vi "Change Desired Temperature.vi"(8 "error in (no error)":cluster{"状态":bool, "代码":i32, "源":string} caption="错误输入（无错误）", 10 "待维持的温度":dbl, 11 "冷却器的控制器输入":refnum<class "Cooler Controller.lvclass">) -> (0 "error out":cluster{"状态":bool, "代码":i32, "源":string} caption="错误输出", 3 "冷却器的控制器输出":refnum<class "Cooler Controller.lvclass">)   [LabVIEW 2013, in "Cooler Controller.lvlib" / "Cooler Controller.lvclass"]
doc: "更改冷却系统需要维持的温度。"
uses:
  Cooler Controller.lvclass
  Cooler Controller.lvclass/Cooler Controller.ctl
  Cooler/Write Desired Temperature Msg/Write Desired Temperature Msg.lvclass/Write Desired Temperature Msg.ctl
  <vilib>/ActorFramework/Message Enqueuer/Message Enqueuer.lvclass/Message Enqueuer.ctl
  <vilib>/ActorFramework/Message Enqueuer/Enqueue.vi
  <vilib>/ActorFramework/Message Priority Queue/Priority Enqueue.vi
  Cooler/Write Desired Temperature Msg/Write Desired Temperature Msg.lvclass
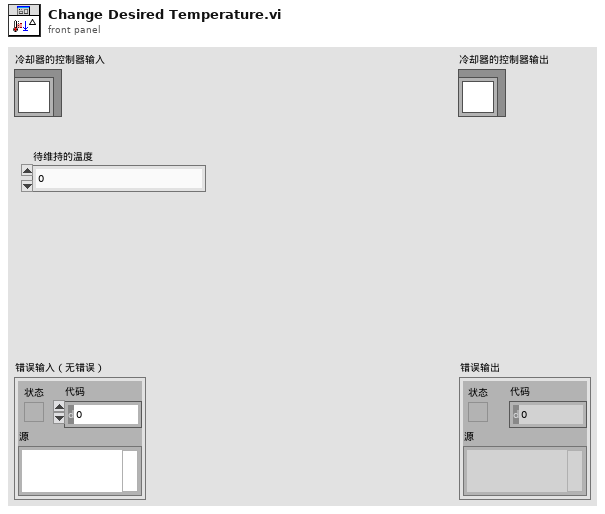
[diagram p1: front panel]
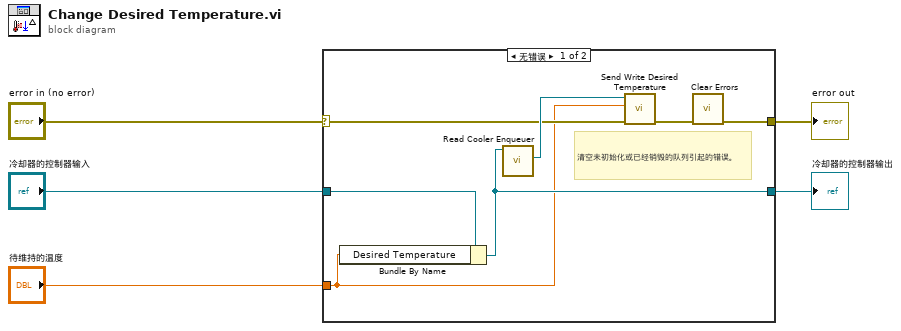
[diagram p0: block diagram]
diagram:
  n1 = case shown="无错误" "error in (no error)" {
    selector: "error in (no error)" -> [w11 w14]
    tunnel: [w6 w14] -> w4
    tunnel: [w9 w13] -> w2
    tunnel: "冷却器的控制器输入" -> [w10 w13]
    tunnel: "待维持的温度" -> [w8 _]
    frame No Error {
      # "清空未初始化或已经销毁的队列引起的错误。"
      n2 = Bundle By Name(cluster=w10, "Desired Temperature"=w8) -> (w9:refnum<class "Cooler Controller.lvclass">)
      n3 = call "Read Cooler Enqueuer.vi"("冷却器控制器"=w9) -> ("冷却器待入队列"=w12:refnum<class "Message Enqueuer.lvclass">)  [unwired: 10 in]
      n4 = call "Send Write Desired Temperature.vi"("error in (no error)"=w11, "待维持的温度"=w8, "消息待入队列"=w12) -> ("error out"=w7:cluster{"状态":bool, "代码":i32, "源":string})  [unwired: 8 in]
      n5 = call <vilib>:"Clear Errors.vi"("error in (no error)"=w7) -> ("error out"=w6:errorcluster)  [unwired: 6 in]
    }
    frame Error {
    }
  }
  "error out" <- w4
  "冷却器的控制器输出" <- w2
